vi "Periodic Tasks.vi"(8 "error in":errorcluster) -> ()   [LabVIEW 2016]
doc: "This VI runs in parallel to other tasks. It can contain as many user-defined periodic loops as you need. These can carry out PID or other sorts of timed response."
uses:
  <vilib>/Rock Robotics/WPI/Utilities/WPI_GetSetVariantRefNum.vi
panel:
  in  "frontleft":bool
  in  "frontright":bool
  in  "backright":bool
  in  "backleft":bool
  in  "power value":dbl
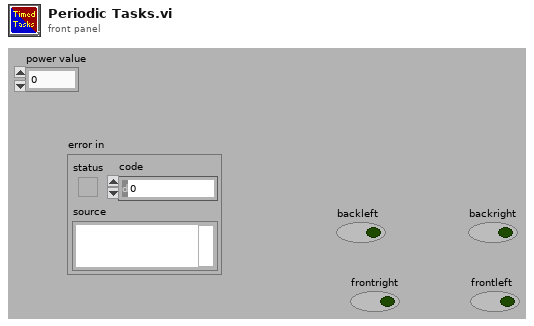
[diagram p1: front panel]
types:
  T1 = typedef "WPI_MotorControlDeviceRef.ctl" = cluster{"DeviceStatus":errorcluster, "Type":T2, "PWM":cluster{"PWM Channel":T3, "DeadBand":T4}, "CAN":cluster{"Device Number":u8, "SetOutput VI Ref":variant, "GetOutput VI Ref":variant, "Enable VI Ref":variant, "Disable VI Ref":variant, "Data":variant}, "Invert":bool}
  T2 = typedef "WPI_MotorControlType.ctl" = enum16{"PWM", "CAN"}
  T3 = typedef "FPGA_DIOPWMChannel.ctl" = enum8{"PWM 0", "PWM 1", "PWM 2", "PWM 3", "PWM 4", "PWM 5", "PWM 6", "PWM 7", "PWM 8", "PWM 9", "PWM MXP 0", "PWM MXP 1", "PWM MXP 2", "PWM MXP 3", "PWM MXP 4", "PWM MXP 5", "PWM MXP 6", "PWM MXP 7", "PWM MXP 8", "PWM MXP 9", "Invalid"}
  T4 = typedef "WPI_PWMDeadband.ctl" = cluster{"Name":string, "maxPositivePwm":i32, "minPositivePwm":i32, "centerPwm":i32, "maxNegativePwm":i32, "minNegativePwm":i32, "angularRange":u16}
  T5 = typedef "WPI_JoystickDevRef.ctl" = cluster{"Device":T6}
  T6 = typedef "WPI_JoystickDeviceEnum.ctl" = enum16{"USB 0", "USB 1", "USB 2", "USB 3", "USB 4", "USB 5"}
  T7 = cluster{"Axes[0]":dbl, "Axes[1]":dbl, "Axes[2]":dbl, "Axes[3]":dbl, "Axes[4]":dbl, "Axes[5]":dbl, "Axes[6]":dbl, "Axes[7]":dbl, "Axes[8]":dbl}
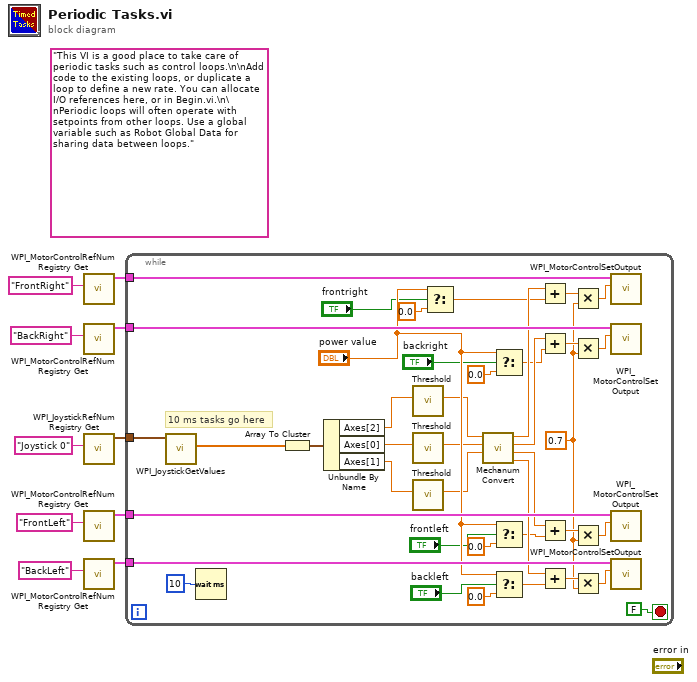
[diagram p0: block diagram]
diagram:
  (unwired) "This VI is a good place to take care of periodic tasks such as control loops.\n\nAdd code to the existing loops, or duplicate a loop to define a new rate. You can allocate I/O references here, or in Begin.vi.\n\nPeriodic loops will often operate with setpoints from other loops. Use a global variable such as Robot Global Data for sharing data between loops."
  n1 = call <vilib>:"WPI_MotorControlRefNum Registry Get.vi"("refnum name"="FrontRight") -> ("MotorControlDevRef"=w3:T1)  [unwired: 9 in, 1 out]
  n2 = call <vilib>:"WPI_MotorControlRefNum Registry Get.vi"("refnum name"="BackRight") -> ("MotorControlDevRef"=w2:T1)  [unwired: 9 in, 1 out]
  n3 = call <vilib>:"WPI_JoystickRefNum Registry Get.vi"("refnum name"="Joystick 0") -> ("JoystickDevRef"=w1:T5)  [unwired: 1 in, 9 out]
  n4 = call <vilib>:"WPI_MotorControlRefNum Registry Get.vi"("refnum name"="FrontLeft") -> ("MotorControlDevRef"=w5:T1)  [unwired: 9 in, 1 out]
  n5 = call <vilib>:"WPI_MotorControlRefNum Registry Get.vi"("refnum name"="BackLeft") -> ("MotorControlDevRef"=w4:T1)  [unwired: 9 in, 1 out]
  n6 = while {
    tunnel: w5 -> [w49]
    tunnel: w4 -> [w48]
    tunnel: w3 -> [w47]
    tunnel: w2 -> [w46]
    tunnel: w1 -> [w45]
    stop <- FALSE stop-if-true
    w11 = 0.7 ("y")
    # "10 ms tasks go here"
    n7 = call <vilib>:"WPI_JoystickGetValues.vi"("JoystickDevRef"=w45) -> ("Axes"=w44:dbl[])  [unwired: 6 in, 4 out]
    n8 = Wait (ms)(milliseconds to wait=u32 10) -> ()  [unwired: 1 out]
    n9 = Array To Cluster(array=w44) -> (cluster=w43:T7)
    n10 = Unbundle By Name(w43) -> ("Axes[2]"=w38:dbl, "Axes[0]"=w37:dbl, "Axes[1]"=w36:dbl)
    n11 = call "Threshold.vi"("Input"=w38) -> ("Output"=w18:dbl)  [unwired: 10 in]
    n12 = call "Threshold.vi"("Input"=w37) -> ("Output"=w17:dbl)  [unwired: 10 in]
    n13 = call "Threshold.vi"("Input"=w36) -> ("Output"=w16:dbl)  [unwired: 10 in]
    n14 = Select(t="power value", s="frontright", f=0.0) -> (s? t:f=w29:dbl)
    n15 = call "Mechanum Convert.vi"("Axes[1]"=w16, "Axes[0]"=w17, "Axes[2]"=w18) -> ("BackLeft"=w42:dbl, "FrontLeft"=w41:dbl, "BackRight"=w40:dbl, "FrontRight"=w39:dbl)  [unwired: 5 in]
    n16 = Select(t="power value", s="backright", f=0.0) -> (s? t:f=w30:dbl)
    n17 = Select(t="power value", s="frontleft", f=0.0) -> (s? t:f=w28:dbl)
    n18 = Select(t="power value", s="backleft", f=0.0) -> (s? t:f=w31:dbl)
    n19 = Add(x=w39, y=w29) -> (x+y=w34:dbl)
    n20 = Add(x=w40, y=w30) -> (x+y=w33:dbl)
    n21 = Add(x=w41, y=w28) -> (x+y=w35:dbl)
    n22 = Add(x=w42, y=w31) -> (x+y=w32:dbl)
    n23 = Multiply(x=w34, y=w11) -> (x*y=w13:dbl)
    n24 = Multiply(x=w33, y=w11) -> (x*y=w12:dbl)
    n25 = Multiply(x=w35, y=w11) -> (x*y=w15:dbl)
    n26 = Multiply(x=w32, y=w11) -> (x*y=w14:dbl)
    n27 = call <vilib>:"WPI_MotorControlSetOutput.vi"("Output"=w13, "MotorControlDevRef"=w47) -> ()  [unwired: 7 in, 3 out]
    n28 = call <vilib>:"WPI_MotorControlSetOutput.vi"("Output"=w12, "MotorControlDevRef"=w46) -> ()  [unwired: 7 in, 3 out]
    n29 = call <vilib>:"WPI_MotorControlSetOutput.vi"("Output"=w15, "MotorControlDevRef"=w49) -> ()  [unwired: 7 in, 3 out]
    n30 = call <vilib>:"WPI_MotorControlSetOutput.vi"("Output"=w14, "MotorControlDevRef"=w48) -> ()  [unwired: 7 in, 3 out]
  }
